vi "TestSetInWave.vi"(8 "error in (no error)":errorcluster) -> (0 "error out":errorcluster)   [LabVIEW 2020]
uses:
  <vilib>/addons/_JKI Toolkits/Caraya/classes/Test/Test.lvclass
  <vilib>/addons/_JKI Toolkits/Caraya/classes/Assert/Assert.lvclass
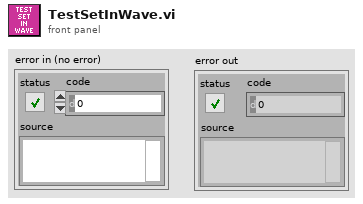
[diagram p1: front panel]
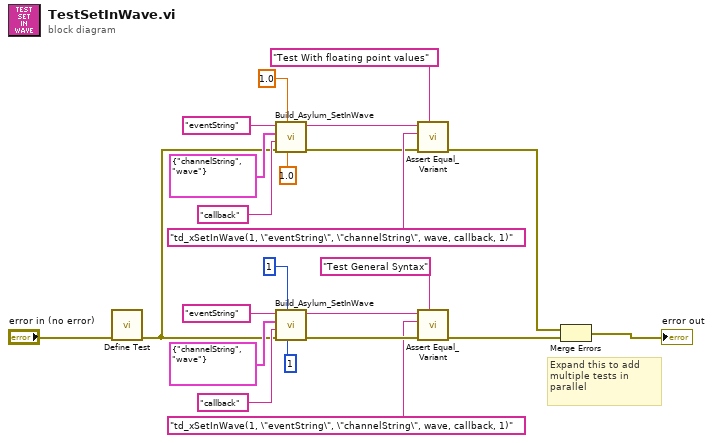
[diagram p0: block diagram]
diagram:
  # "Expand this to add multiple tests in parallel"
  n1 = call <vilib>:"Define Test.vi"("error in (no error)"="error in (no error)") -> ("error out"=w2:errorcluster)  [unwired: 10 in]
  n2 = call "Build_Asylum_SetInWave.vi"("decimation"=1.0, "whichBank"=1.0, "error in (no error)"=w2, "callback"="callback", "Wave"=cluster{"channelString":string, "wave":string} {"channelString"="channelString", "wave"="wave"}, "eventString"="eventString") -> ("error out"=w4:errorcluster, "Command"=w5:string)  [unwired: 4 in]
  n3 = call "Build_Asylum_SetInWave.vi"("decimation"=1, "whichBank"=1, "error in (no error)"=w2, "callback"="callback", "Wave"=cluster{"channelString":string, "wave":string} {"channelString"="channelString", "wave"="wave"}, "eventString"="eventString") -> ("error out"=w19:errorcluster, "Command"=w18:string)  [unwired: 4 in]
  n4 = call <vilib>:"Assert Equal_Variant.vi"("Label"="Test With floating point values", "error in (no error)"=w4, "Y"="td_xSetInWave(1, \"eventString\", \"channelString\", wave, callback, 1)", "X"=w5) -> ("error out"=w1:errorcluster)  [unwired: 7 in]
  n5 = call <vilib>:"Assert Equal_Variant.vi"("Label"="Test General Syntax", "error in (no error)"=w19, "Y"="td_xSetInWave(1, \"eventString\", \"channelString\", wave, callback, 1)", "X"=w18) -> ("error out"=w21:errorcluster)  [unwired: 7 in]
  n6 = Merge Errors(w1, w21) -> (→"error out":errorcluster)
